vi "Step Average.vi"(8 "error in (no error)":errorcluster, 9 "width (c)":dbl, 10 "position (b)":dbl, 11 "Scale":dbl[](array[numeric])) -> (0 "error out":errorcluster, 1 "End":dbl, 2 "Start":dbl, 3 "Averaged Result":dbl[](array[numeric]))   [LabVIEW 2019, in "graph_utilities.lvclass"]
uses:
  graph_utilities.lvclass
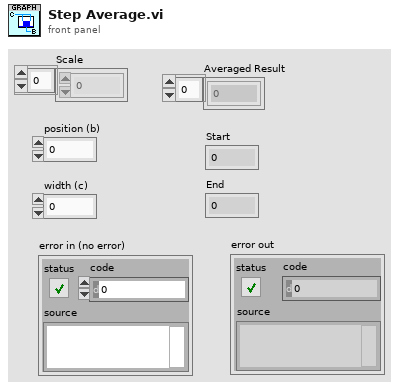
[diagram p1: front panel]
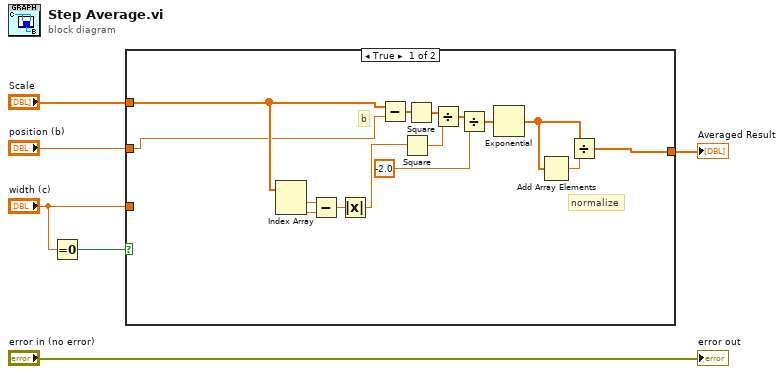
[diagram p0: block diagram]
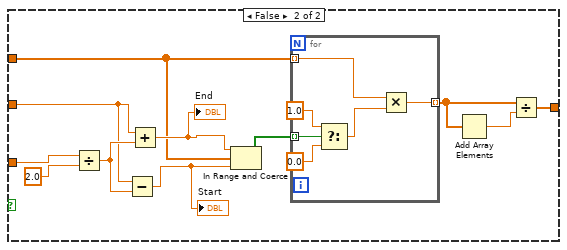
[diagram p2: hidden frame]
diagram:
  n1 = Equal To 0?(x="width (c)") -> (x = 0?=w1:bool)
  n2 = case shown="True" w1 {
    tunnel: [w7 w28] -> w6
    tunnel: "Scale" -> [w10 w23]
    tunnel: "position (b)" -> [w9 w27]
    tunnel: "width (c)" -> [_ w26]
    frame True {
      # "normalize"
      # "b"
      n3 = Index Array(array=w10) -> (element #1=w13:dbl, element #2=w12:dbl)  [unwired: 2 in]
      n4 = Subtract(x=w13, y=w12) -> (x-y=w11:dbl)
      n5 = Absolute Value(x=w11) -> (abs(x)=w8:dbl)
      n6 = Subtract(x=w10, y=w9) -> (x-y=w14:dbl[])
      n7 = Square(x=w8) -> (x^2=w16:dbl)
      n8 = Square(x=w14) -> (x^2=w15:dbl[])
      n9 = Divide(x=w15, y=w16) -> (x/y=w17:dbl[])
      n10 = Divide(x=w17, y=-2.0 ("value")) -> (x/y=w19:dbl[])
      n11 = Exponential(1:w19) -> (0:w21:dbl[])
      n12 = Add Array Elements(numeric array=w21) -> (sum=w20:dbl)
      n13 = Divide(x=w21, y=w20) -> (x/y=w7:dbl[])
    }
    frame False {
      n14 = Divide(x=w26, y=2.0) -> (x/y=w31:dbl)
      n15 = Subtract(x=w27, y=w31) -> (x-y=w25:dbl)
      "Start" <- w25
      n16 = Add(x=w27, y=w31) -> (x+y=w24:dbl)
      "End" <- w24
      n17 = In Range and Coerce(upper limit=w24, x=w23, lower limit=w25) -> (In Range?=w30:bool[])  [unwired: 1 out]
      n18 = for {
        tunnel: w30 -> [w38] mode=indexing
        tunnel: w23 -> [w35] mode=indexing
        tunnel: [w33] -> w22 mode=indexing
        n19 = Select(t=1.0, s=w38, f=0.0) -> (s? t:f=w34:dbl)
        n20 = Multiply(x=w35, y=w34) -> (x*y=w33:dbl)
      }
      n21 = Add Array Elements(numeric array=w22) -> (sum=w29:dbl)
      n22 = Divide(x=w22, y=w29) -> (x/y=w28:dbl[])
    }
  }
  "Averaged Result" <- w6
  "error out" <- "error in (no error)"
